vi "spi_interface_kyles.vi"() -> ()   [LabVIEW 2012]
uses:
  <vilib>/rvi/DataTransferAndStorage/Container/Common/niFpgaContainerMetaDataKey.ctl
  <vilib>/rvi/DataTransferAndStorage/Container/Common/niFpgaContainerState.ctl
  <vilib>/rvi/DataTransferAndStorage/Container/Common/niFpgaDataTypeControl.ctl
  <vilib>/rvi/DataTransferAndStorage/Container/Common/niFpgaContainerImplementationControl.ctl
  <vilib>/rvi/DataTransferAndStorage/Container/Common/niFpgaContainerArbitrationOptionsControl.ctl
  <vilib>/rvi/DataTransferAndStorage/Container/Common/niFpgaTransferTypeControl.ctl
  <vilib>/rvi/DataTransferAndStorage/Container/Common/niFpgaContainerInitializationParameters.ctl
  <vilib>/rvi/Memory/Memory_Types/niFpgaMemoryInterfaceConfiguration.ctl
  <vilib>/rvi/FIFO/Fifo_Types/niFpgaFifoControlLogicControl.ctl
  Controls/FPGA SPI_SPI Loop State.ctl
  <vilib>/rvi/DataTransferAndStorage/Container/Common/niFpgaContainerGetUniqueNameForEmu.vi
  <vilib>/rvi/DataTransferAndStorage/Container/Common/niFpgaContainerSetEmuInfo.vi
  <vilib>/rvi/eio/common/nirviEmuReportErrorAndStop.vi
  <vilib>/rvi/eio/common/nirviEmuTemplateMethod_errors.vi
  <vilib>/rvi/Emulation/niFpgaSctlEmulationGetInTimedLoop.vi
  <vilib>/rvi/FIFO/Fifo_Resource/nirvififoEmulationSetSize.vi
  <vilib>/rvi/errors/niFpgaSetErrorForExecOnDevCompSimple.vi
  <vilib>/rvi/Emulation/niFpgaSctlEmulationFifoFullMgr.vi
  <vilib>/rvi/Emulation/niFpgaSctlEmulationResourceMgr.vi
  <vilib>/rvi/Emulation/niFpgaSctlEmulationGlobalWrite.vi
  <vilib>/rvi/LocalResourceManager/LocalResourceManager.xnode
  <vilib>/eio/EIOMethodNode/EIOMethodNode.xnode
  <vilib>/eio/EIONode/EIONode.xnode
  <vilib>/rvi/DataTransferAndStorage/Container/XNode/niFpgaContainer.xnode
  <vilib>/rvi/FIFO/Fifo_Resource/nirvififoEmulationWrite.vi
  <vilib>/rvi/FIFO/Fifo_Resource/nirvififoEmulationRead.vi
panel:
  in  "CS-read Delay":u8=1
  in  "CS-write Delay":u8=25
  in  "CS-set Delay":u8=2
  in  "Clock Delay(uS)":u32=2
  in  "Read?":bool
  in  "Start SPI":bool
  out "Data Out":u8[](array[numeric]) format="%.0x"
  in  "Data In":u8[](array[numeric])=[0, 0] format="%.0x"
  in  "FPGA IO":T1={"SCLK"="DIO18", "CS_1"="DIO16", "MOSI"="DIO26", "MISO"="DIO25"}
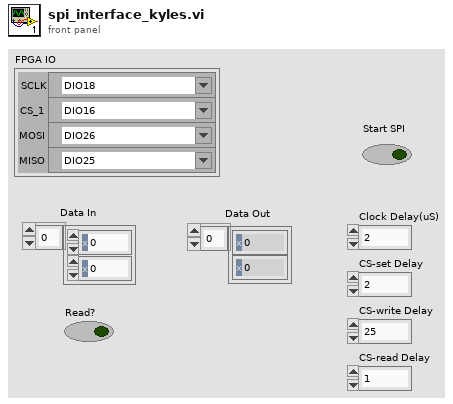
[diagram p1: front panel]
types:
  T1 = cluster{"SCLK":refnum<k21>, "CS_1":refnum<k21>, "MOSI":refnum<k21>, "MISO":refnum<k21>}
  T2 = typedef "FPGA SPI_SPI Loop State.ctl" = enum8{"Initialize", "Set CS", "Read From FIFO", "Send Byte", "Write to FIFO", "Reset CS", "Read Delay"}
  T3 = cluster{"MOSI":bool[], "MISO":bool[], "Read?":bool}
  T4 = cluster{"Next State":T2, "Total Bytes":u16, "Future State":T2, "Read Wait":u32, "CS Reset Wait":u32, "Byte Count":u16}
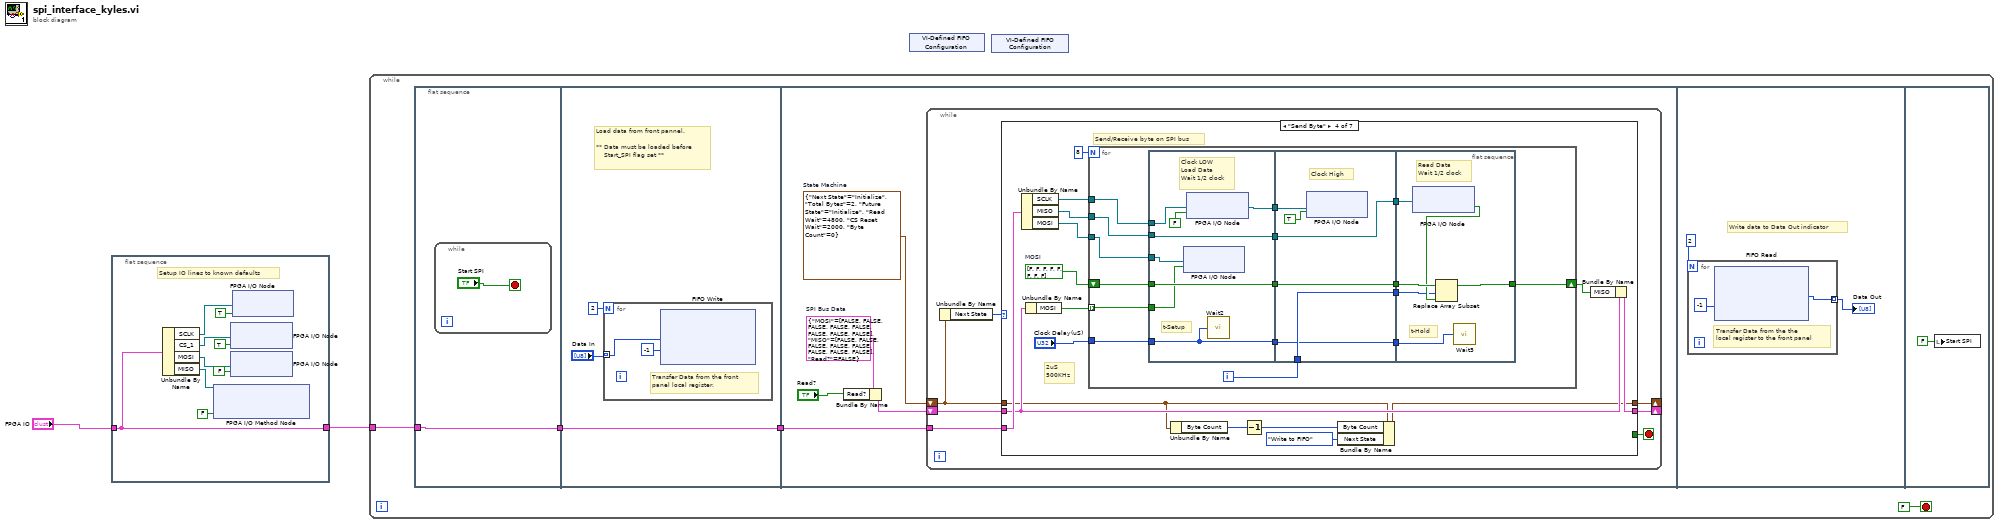
[diagram p0: block diagram]
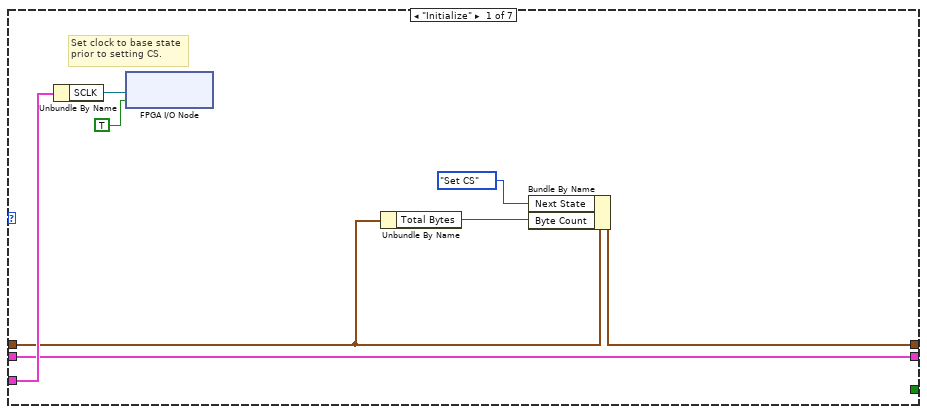
[diagram p2: hidden frame]
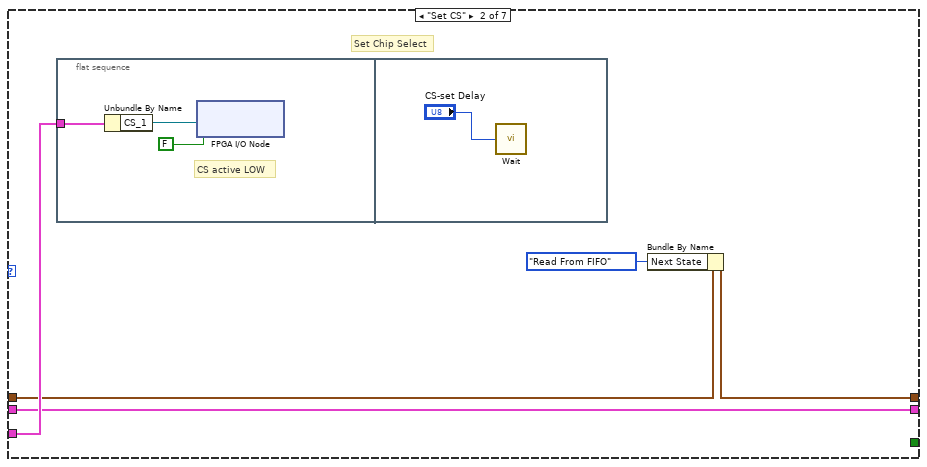
[diagram p3: hidden frame]
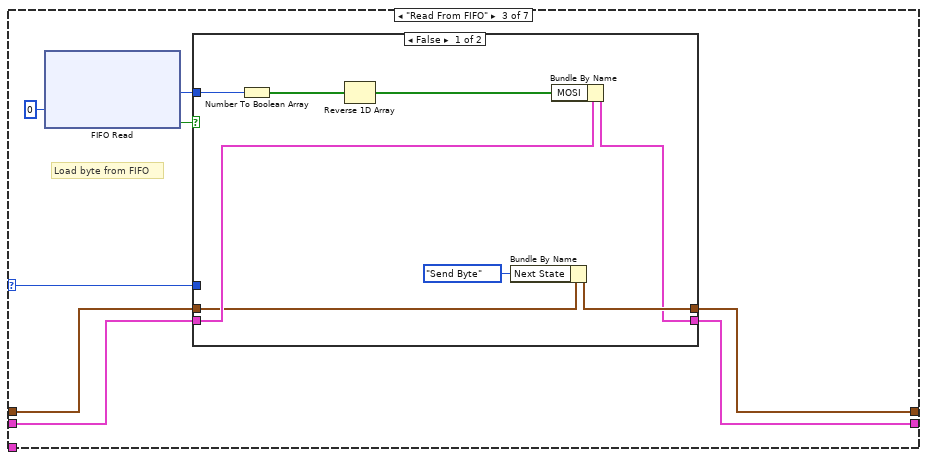
[diagram p4: hidden frame]
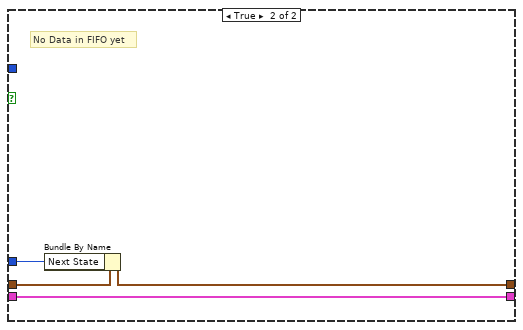
[diagram p5: hidden frame]
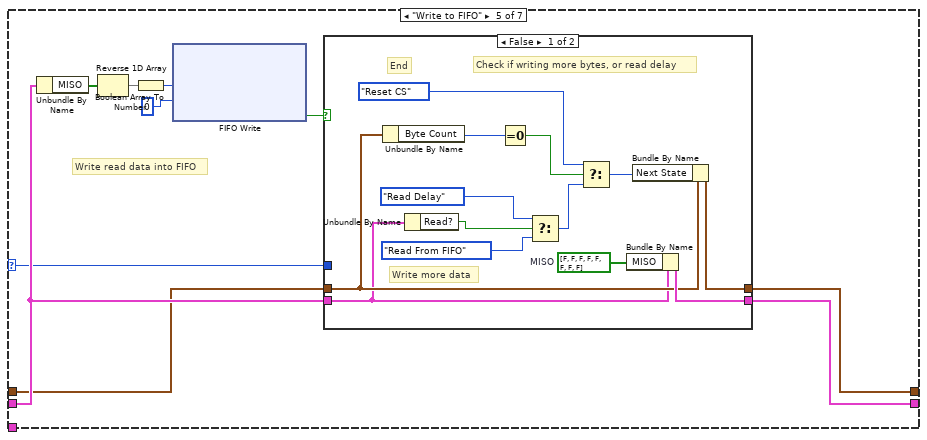
[diagram p6: hidden frame]
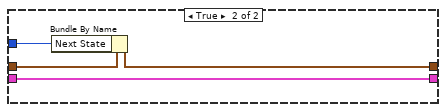
[diagram p7: hidden frame]
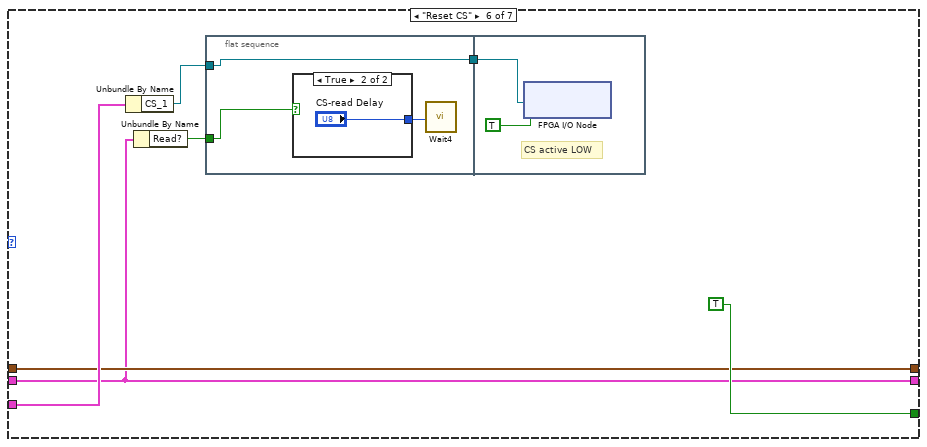
[diagram p8: hidden frame]
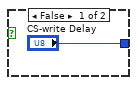
[diagram p9: hidden frame]
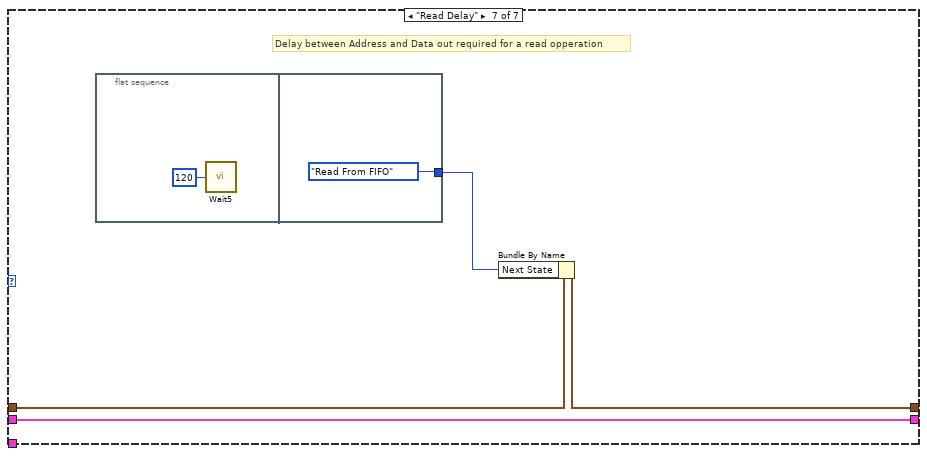
[diagram p10: hidden frame]
diagram:
  n1 = flat-sequence {
    tunnel: [w3] -> w2
    tunnel: "FPGA IO" -> [w3]
    frame #0 {
      # "Setup IO lines to known defaults"
      n2 = Unbundle By Name(w3) -> ("SCLK"=w11:refnum<k21>, "CS_1"=w10:refnum<k21>, "MOSI"=w9:refnum<k21>, "MISO"=w4:refnum<k21>)
      n3 = xnode "FPGA I/O Method Node"("FPGA I/O In"=w4, "Enable"=FALSE) -> ()  [unwired: 1 out]
      n4 = xnode "FPGA I/O Node"("I/O Item"=TRUE, "FPGA I/O In"=w10) -> ()  [unwired: 1 out]
      n5 = xnode "FPGA I/O Node"("I/O Item"=FALSE, "FPGA I/O In"=w9) -> ()  [unwired: 1 out]
      n6 = xnode "FPGA I/O Node"("I/O Item"=TRUE, "FPGA I/O In"=w11) -> ()  [unwired: 1 out]
    }
  }
  n7 = while {
    tunnel: w2 -> [w14]
    stop <- FALSE stop-if-true
    n8 = flat-sequence {
      tunnel: w14 -> [w16]
      tunnel: [w16] -> w12
      tunnel: [w18] -> w13
      tunnel: w12 -> [w18]
      tunnel: w13 -> [w23]
      frame #0 {
        n9 = while {
          stop <- "Start SPI" stop-if-true
        }
      }
      frame #1 {
        # "Load data from front pannel.\n\n** Data must be loaded before \n    Start_SPI flag set **"
        n10 = for {
          N: 2 -> [_]
          tunnel: "Data In" -> [w21] mode=indexing
          # "Transfer Data from the front \npanel local register."
          n11 = xnode ("FIFO Write")("Element"=w21, "Timeout"=-1) -> ()  [unwired: 1 in, 2 out]
        }
      }
      frame #2 {
        w25 = T3 {"MOSI"=[FALSE, FALSE, FALSE, FALSE, FALSE, FALSE, FALSE, FALSE], "MISO"=[FALSE, FALSE, FALSE, FALSE, FALSE, FALSE, FALSE, FALSE], "Read?"=FALSE}  # SPI Bus Data
        w24 = T4 {"Next State"=enum."Initialize", "Total Bytes"=2, "Future State"=enum."Initialize", "Read Wait"=4800, "CS Reset Wait"=2000, "Byte Count"=0}  # State Machine
        n12 = Bundle By Name(cluster=w25, "Read?"="Read?") -> (w27:T3)
        n13 = while {
          shift-right: [w34] -> _
          shift-left: w24 -> [w33]
          tunnel: w23 -> [w29]
          shift-right: [w30] -> _
          shift-left: w27 -> [w31]
          stop <- w28 stop-if-true
          n14 = Unbundle By Name(w33) -> ("Next State"=w32:T2)
          n15 = case shown="\"Send Byte\"" w32 {
            selector: w32 -> [_ _ w52 _ w126 _ _]
            tunnel: w33 -> [w36 w45 w54 w72 w125 w154 w168]
            tunnel: [w40 w47 w57 w80 w131 w154 w166] -> w34
            tunnel: w31 -> [w37 w44 w55 w82 w129 w152 w167]
            tunnel: [w37 w44 w56 w81 w128 w152 w167] -> w30
            tunnel: w29 -> [w42 w46 _ w87 _ w157 _]
            tunnel: [_ _ _ _ _ TRUE _] -> w28
            frame "Initialize" {
              # "Set clock to base state\nprior to setting CS."
              n16 = Unbundle By Name(w42) -> ("SCLK"=w41:refnum<k21>)
              n17 = xnode "FPGA I/O Node"("I/O Item"=TRUE, "FPGA I/O In"=w41) -> ()  [unwired: 1 out]
              n18 = Unbundle By Name(w36) -> ("Total Bytes"=w35:u16)
              n19 = Bundle By Name(cluster=w36, "Next State"=FPGA_SPI_SPI_Loop_State."Set CS", "Byte Count"=w35) -> (w40:T4)
            }
            frame "Set CS" {
              # "Set Chip Select"
              n20 = flat-sequence {
                tunnel: w46 -> [w50]
                frame #0 {
                  # "CS active LOW"
                  n21 = Unbundle By Name(w50) -> ("CS_1"=w49:refnum<k21>)
                  n22 = xnode "FPGA I/O Node"("I/O Item"=FALSE, "FPGA I/O In"=w49) -> ()  [unwired: 1 out]
                }
                frame #1 {
                  n23 = call "Wait"("Count(uSec)"="CS-set Delay") -> ()  [unwired: 1 out]
                }
              }
              n24 = Bundle By Name(cluster=w45, "Next State"=FPGA_SPI_SPI_Loop_State."Read From FIFO") -> (w47:T4)
            }
            frame "Read From FIFO" {
              # "Load byte from FIFO"
              n25 = xnode ("FIFO Read")("Timeout"=0) -> ("Element"=w58:u8, "Timed Out?"=w53:bool)  [unwired: 1 in, 1 out]
              n26 = case shown="False" w53 {
                tunnel: w58 -> [w67 _]
                tunnel: [w66 w68] -> w57
                tunnel: [w65 w71] -> w56
                tunnel: w55 -> [w64 w71]
                tunnel: w54 -> [w62 w69]
                tunnel: w52 -> [_ w70]
                frame False {
                  n27 = Number To Boolean Array(number=w67) -> (Boolean array=w63:bool[])
                  n28 = Reverse 1D Array(array=w63) -> (reversed array=w60:bool[])
                  n29 = Bundle By Name(cluster=w62, "Next State"=FPGA_SPI_SPI_Loop_State."Send Byte") -> (w66:T4)
                  n30 = Bundle By Name(cluster=w64, "MOSI"=w60) -> (w65:T3)
                }
                frame True {
                  # "No Data in FIFO yet"
                  n31 = Bundle By Name(cluster=w69, "Next State"=w70) -> (w68:T4)
                }
              }
            }
            frame "Send Byte" {
              w77 = bool[] [FALSE, FALSE, FALSE, FALSE, FALSE, FALSE, FALSE, FALSE]  # MOSI
              # "2uS\n500KHz"
              # "Send/Receive byte on SPI bus"
              n32 = Unbundle By Name(w87) -> ("SCLK"=w86:refnum<k21>, "MISO"=w84:refnum<k21>, "MOSI"=w85:refnum<k21>)
              n33 = Unbundle By Name(w82) -> ("MOSI"=w73:bool[])
              n34 = for {
                N: 8 -> [_]
                tunnel: w73 -> [w103] mode=indexing
                tunnel: w86 -> [w102]
                tunnel: w85 -> [w101]
                tunnel: w84 -> [w100]
                tunnel: "Clock Delay(uS)" -> [w99]
                shift-right: [w93] -> w76
                shift-left: w77 -> [w97]
                i -> [w96]
                n35 = flat-sequence {
                  tunnel: w103 -> [w104]
                  tunnel: w102 -> [w111]
                  tunnel: w101 -> [w105]
                  tunnel: w100 -> [w109]
                  tunnel: [w109] -> w91
                  tunnel: [w108] -> w90
                  tunnel: w99 -> [w106]
                  tunnel: [w106] -> w89
                  tunnel: [w107] -> w88
                  tunnel: w97 -> [w107]
                  tunnel: [w112] -> w98
                  tunnel: w96 -> [w113]
                  tunnel: [w115] -> w95
                  tunnel: [w114] -> w94
                  tunnel: [w113] -> w92
                  tunnel: w88 -> [w114]
                  tunnel: w89 -> [w112]
                  tunnel: w90 -> [w116]
                  tunnel: w91 -> [w115]
                  tunnel: w98 -> [w123]
                  tunnel: w95 -> [w122]
                  tunnel: w94 -> [w121]
                  tunnel: [w120] -> w93
                  tunnel: w92 -> [w118]
                  frame #0 {
                    # "t-Setup"
                    # "Clock LOW\nLoad Data\nWait 1/2 clock"
                    n36 = xnode "FPGA I/O Node"("I/O Item"=w104, "FPGA I/O In"=w105) -> ()  [unwired: 1 out]
                    n37 = xnode "FPGA I/O Node"("I/O Item"=FALSE, "FPGA I/O In"=w111) -> ("FPGA I/O Out"=w108:refnum<k21>)
                    n38 = call "Wait2"("Count(uSec)"=w106) -> ()  [unwired: 1 out]
                  }
                  frame #1 {
                    # "Clock High"
                    n39 = xnode "FPGA I/O Node"("I/O Item"=TRUE, "FPGA I/O In"=w116) -> ()  [unwired: 1 out]
                  }
                  frame #2 {
                    # "Read Data\nWait 1/2 clock"
                    # "t-Hold"
                    n40 = xnode "FPGA I/O Node"("FPGA I/O In"=w122) -> ("I/O Item"=w119:bool)  [unwired: 1 out]
                    n41 = Replace Array Subset(array=w121, new element=w119, index=w118) -> (w120:bool[])
                    n42 = call "Wait3"("Count(uSec)"=w123) -> ()  [unwired: 1 out]
                  }
                }
              }
              n43 = Unbundle By Name(w72) -> ("Byte Count"=w75:u16)
              n44 = Decrement(x=w75) -> (x-1=w74:u16)
              n45 = Bundle By Name(cluster=w72, "Byte Count"=w74, "Next State"=FPGA_SPI_SPI_Loop_State."Write to FIFO") -> (w80:T4)
              n46 = Bundle By Name(cluster=w82, "MISO"=w76) -> (w81:T3)
            }
            frame "Write to FIFO" {
              # "Write read data into FIFO"
              n47 = Unbundle By Name(w129) -> ("MISO"=w133:bool[])
              n48 = Reverse 1D Array(array=w133) -> (reversed array=w124:bool[])
              n49 = Boolean Array To Number(Boolean array=w124) -> (number=w132:u8)
              n50 = xnode ("FIFO Write")("Element"=w132, "Timeout"=0) -> ("Timed Out?"=w127:bool)  [unwired: 1 in, 1 out]
              n51 = case shown="False" w127 {
                tunnel: [w146 w148] -> w131
                tunnel: w125 -> [w140 w149]
                tunnel: w129 -> [w135 w150]
                tunnel: [w142 w150] -> w128
                tunnel: w126 -> [_ w147]
                frame False {
                  w143 = bool[] [FALSE, FALSE, FALSE, FALSE, FALSE, FALSE, FALSE, FALSE]  # MISO
                  # "Check if writing more bytes, or read delay"
                  # "Write more data"
                  # "End"
                  n52 = Unbundle By Name(w140) -> ("Byte Count"=w138:u16)
                  n53 = Unbundle By Name(w135) -> ("Read?"=w134:bool)
                  n54 = Equal To 0?(x=w138) -> (x = 0?=w139:bool)
                  n55 = Select(t=FPGA_SPI_SPI_Loop_State."Read Delay", s=w134, f=FPGA_SPI_SPI_Loop_State."Read From FIFO" ("Next State")) -> (s? t:f=w137:T2)
                  n56 = Select(t=FPGA_SPI_SPI_Loop_State."Reset CS" ("Next State"), s=w139, f=w137) -> (s? t:f=w144:T2)
                  n57 = Bundle By Name(cluster=w135, "MISO"=w143) -> (w142:T3)
                  n58 = Bundle By Name(cluster=w140, "Next State"=w144) -> (w146:T4)
                }
                frame True {
                  n59 = Bundle By Name(cluster=w149, "Next State"=w147) -> (w148:T4)
                }
              }
            }
            frame "Reset CS" {
              n60 = Unbundle By Name(w157) -> ("CS_1"=w155:refnum<k21>)
              n61 = Unbundle By Name(w152) -> ("Read?"=w151:bool)
              n62 = flat-sequence {
                tunnel: w155 -> [w160]
                tunnel: [w160] -> w153
                tunnel: w151 -> [w158]
                tunnel: w153 -> [w163]
                frame #0 {
                  n63 = case shown="True" w158 {
                    tunnel: ["CS-write Delay" "CS-read Delay"] -> w159
                    frame False {
                    }
                    frame True {
                    }
                  }
                  n64 = call "Wait4"("Count(uSec)"=w159) -> ()  [unwired: 1 out]
                }
                frame #1 {
                  # "CS active LOW"
                  n65 = xnode "FPGA I/O Node"("I/O Item"=TRUE, "FPGA I/O In"=w163) -> ()  [unwired: 1 out]
                }
              }
            }
            frame "Read Delay" {
              # "Delay between Address and Data out required for a read opperation"
              n66 = flat-sequence {
                tunnel: [FPGA_SPI_SPI_Loop_State."Read From FIFO" ("Next State")] -> w165
                frame #0 {
                  n67 = call "Wait5"("Count(uSec)"=u16 120) -> ()  [unwired: 1 out]
                }
                frame #1 {
                }
              }
              n68 = Bundle By Name(cluster=w168, "Next State"=w165) -> (w166:T4)
            }
          }
        }
      }
      frame #3 {
        # "Write data to Data Out indicator"
        n69 = for {
          N: 2 -> [_]
          tunnel: [w173] -> w172 mode=indexing
          # "Transfer Data from the the \nlocal register to the front panel"
          n70 = xnode ("FIFO Read")("Timeout"=-1) -> ("Element"=w173:u8)  [unwired: 1 in, 2 out]
        }
        "Data Out" <- w172
      }
      frame #4 {
        n71 = local write "Start SPI"(FALSE ("Start SPI")) -> ()
      }
    }
  }
  n72 = xnode "VI-Defined FIFO Configuration"() -> ()  [unwired: 1 out]
  n73 = xnode "VI-Defined FIFO Configuration"() -> ()  [unwired: 1 out]
